vi "Func-엑셀 데이터를 그래프로 출력.vi"() -> ()   [LabVIEW 2015] (continued)
65\t66.118\n65\t65\t66.122\n65\t65\t66.121\n65\t65\t66.127\n65\t65\t66.131\n65\t65\t66.133\n65\t65\t66.137\n65\t65\t66.142\n65\t65\t66.146\n65\t65\t66.148\n65\t65\t66.151\n65\t65\t66.159\n65\t65\t66.161\n65\t65\t66.172\n65\t65\t66.18\n65\t65\t66.186\n65\t65\t66.193\n65\t65\t66.193\n65\t65\t66.2\n65\t65\t66.203\n65\t65\t66.207\n65\t65\t66.213\n65\t65\t66.22\n65\t65\t66.229\n65\t65\t66.235\n65\t65\t66.24\n65\t65\t66.241\n65\t65\t66.25\n65\t65\t66.253\n65\t65\t66.255\n65\t65\t66.258\n65\t65\t66.26\n65\t65\t66.269\n65\t65\t66.273\n65\t65\t66.275\n65\t65\t66.28\n65\t65\t66.287\n65\t65\t66.292\n65\t65\t66.293\n65\t65\t66.298\n65\t65\t66.306\n65\t65\t66.312\n65\t65\t66.318\n65\t65\t66.323\n65\t65\t66.334\n65\t65\t66.34\n65\t65\t66.345\n65\t65\t66.355\n65\t65\t66.36\n65\t65\t66.363\n65\t65\t66.37\n65\t65\t66.37\n65\t65\t66.371\n65\t65\t66.371\n65\t65\t66.377\n65\t65\t66.384\n65\t65\t66.388\n65\t65\t66.393\n65\t65\t66.4\n65\t65\t66.405\n65\t65\t66.407\n65\t65\t66.409\n65\t65\t66.416\n65\t65\t66.424\n65\t65\t66.427\n65\t65\t66.436\n65\t65\t66.44\n65\t65\t66.444\n65\t65\t66.446\n65\t65\t66.448\n65\t65\t66.452\n65\t65\t66.458\n65\t65\t66.463\n65\t65\t66.471\n65\t65\t66.475\n65\t65\t66.484\n65\t65\t66.493\n65\t65\t66.497\n65\t65\t66.506\n65\t65\t66.516\n65\t65\t66.522\n65\t65\t66.525\n65\t65\t66.527\n65\t65\t66.532\n65\t65\t66.532\n65\t65\t66.532\n65\t65\t66.535\n65\t65\t66.545\n65\t65\t66.546\n65\t65\t66.548\n65\t65\t66.55\n65\t65\t66.56\n65\t65\t66.568\n65\t65\t66.571\n65\t65\t66.577\n65\t65\t66.586\n65\t65\t66.591\n65\t65\t66.592\n65\t65\t66.593\n65\t65\t66.597\n65\t65\t66.599\n65\t65\t66.601\n65\t65\t66.609\n65\t65\t66.611\n65\t65\t66.614\n65\t65\t66.619\n65\t65\t66.624\n65\t65\t66.627\n65\t65\t66.629\n65\t65\t66.635\n65\t65\t66.641\n65\t65\t66.645\n65\t65\t66.649\n65\t65\t66.66\n65\t65\t66.666\n65\t65\t66.668\n65\t65\t66.673\n65\t65\t66.68\n65\t65\t66.687\n65\t65\t66.694\n65\t65\t66.699\n65\t65\t66.707\n65\t65\t66.713\n65\t65\t66.717\n65\t65\t66.724\n65\t65\t66.723\n65\t65\t66.73\n65\t65\t66.73\n65\t65\t66.733\n65\t65\t66.736\n65\t65\t66.741\n65\t65\t66.746\n65\t65\t66.747\n65\t65\t66.758\n65\t65\t66.761\n65\t65\t66.761\n65\t65\t66.764\n65\t65\t66.766\n65\t65\t66.773\n65\t65\t66.779\n65\t65\t66.783\n65\t65\t66.79\n65\t65\t66.798\n65\t65\t66.802\n65\t65\t66.804\n65\t65\t66.807\n65\t65\t66.813\n65\t65\t66.818\n65\t65\t66.823\n65\t65\t66.825\n65\t65\t66.827\n65\t65\t66.834\n65\t65\t66.835\n65\t65\t66.84\n65\t65\t66.846\n65\t65\t66.852\n65\t65\t66.862\n65\t65\t66.866\n65\t65\t66.872\n65\t65\t66.879\n65\t65\t66.879\n65\t65\t66.884\n65\t65\t66.891\n65\t65\t66.893\n65\t65\t66.898\n65\t65\t66.9\n65\t65\t66.906\n65\t65\t66.909\n65\t65\t66.909\n65\t65\t66.914\n65\t65\t66.918\n65\t65\t66.925\n65\t65\t66.93\n65\t65\t66.934\n65\t65\t66.939\n65\t65\t66.943\n65\t65\t66.946\n65\t65\t66.948\n65\t65\t66.952\n65\t65\t66.955\n65\t65\t66.958\n65\t65\t66.963\n65\t65\t66.971\n65\t65\t66.976\n65\t65\t66.977\n65\t65\t66.984\n65\t65\t66.988\n65\t65\t66.988\n65\t65\t66.993\n65\t65\t66.998\n65\t65\t67.005\n65\t65\t67.014\n65\t65\t67.021\n65\t65\t67.025\n65\t65\t67.028\n65\t65\t67.029\n65\t65\t67.029\n65\t65\t67.031\n65\t65\t67.033\n65\t65\t67.043\n65\t65\t67.049\n65\t65\t67.05\n65\t65\t67.058\n65\t65\t67.064\n65\t65\t67.069\n65\t65\t67.074\n65\t65\t67.078\n65\t65\t67.087\n65\t65\t67.09\n65\t65\t67.091\n65\t65\t67.091\n65\t65\t67.091\n65\t65\t67.091\n65\t65\t67.093\n65\t65\t67.101\n65\t65\t67.104\n65\t65\t67.113\n65\t65\t67.118\n65\t65\t67.126\n65\t65\t67.129\n65\t65\t67.13\n65\t65\t67.136\n65\t65\t67.139\n65\t65\t67.147\n65\t65\t67.148\n65\t65\t67.155\n65\t65\t67.162\n65\t65\t67.166\n65\t65\t67.175\n65\t65\t67.179\n65\t65\t67.184\n65\t65\t67.187\n65\t65\t67.189\n65\t65\t67.19\n65\t65\t67.191\n65\t65\t67.194\n65\t65\t67.197\n65\t65\t67.204\n65\t65\t67.209\n65\t65\t67.216\n65\t65\t67.221\n65\t65\t67.224\n65\t65\t67.231\n65\t65\t67.232\n65\t65\t67.234\n65\t65\t67.236\n65\t65\t67.239\n65\t65\t67.243\n65\t65\t67.243\n65\t65\t67.248\n65\t65\t67.254\n65\t65\t67.262\n65\t65\t67.264\n65\t65\t67.268\n65\t65\t67.28\n65\t65\t67.285\n65\t65\t67.289\n65\t65\t67.292\n65\t65\t67.298\n65\t65\t67.304\n65\t65\t67.303\n65\t65\t67.308\n65\t65\t67.311\n65\t65\t67.312\n65\t65\t67.317\n65\t65\t67.318\n65\t65\t67.326\n65\t65\t67.332\n65\t65\t67.338\n65\t65\t67.342\n65\t65\t67.347\n65\t65\t67.353\n65\t65\t67.352\n65\t65\t67.352\n65\t65\t67.352\n65\t65\t67.356\n65\t65\t67.357\n65\t65\t67.36\n65\t65\t67.363\n65\t65\t67.372\n65\t65\t67.377\n65\t65\t67.382\n65\t65\t67.388\n65\t65\t67.391\n65\t65\t67.396\n65\t65\t67.399\n65\t65\t67.399\n65\t65\t67.4\n65\t65\t67.406\n65\t65\t67.412\n65\t65\t67.414\n65\t65\t67.417\n65\t65\t67.423\n65\t65\t67.428\n65\t65\t67.429\n65\t65\t67.433\n65\t65\t67.437\n65\t65\t67.445\n65\t65\t67.448\n65\t65\t67.451\n65\t65\t67.454\n65\t65\t67.456\n65\t65\t67.458\n65\t65\t67.458\n65\t65\t67.461\n65\t65\t67.47\n65\t65\t67.475\n65\t65\t67.479\n65\t65\t67.48\n65\t65\t67.486\n65\t65\t67.489\n65\t65\t67.495\n65\t65\t67.498\n65\t65\t67.504\n65\t65\t67.508\n65\t65\t67.513\n65\t65\t67.515\n65\t65\t67.52\n65\t65\t67.52\n65\t65\t67.516\n65\t65\t67.523\n65\t65\t67.525\n65\t65\t67.526\n65\t65\t67.528\n65\t65\t67.533\n65\t65\t67.543\n65\t65\t67.549\n65\t65\t67.554\n65\t65\t67.559\n65\t65\t67.563\n65\t65\t67.564\n65\t65\t67.565\n65\t65\t67.567\n65\t65\t67.571\n65\t65\t67.58\n65\t65\t67.583\n65\t65\t67.588\n65\t65\t67.594\n65\t65\t67.6\n65\t65\t67.599\n65\t65\t67.6\n65\t65\t67.603\n65\t65\t67.61\n65\t65\t67.613\n65\t65\t67.613\n65\t65\t67.62\n65\t65\t67.62\n65\t65\t67.624\n65\t65\t67.631\n65\t65\t67.638\n65\t65\t67.642\n65\t65\t67.646\n65\t65\t67.65\n65\t65\t67.654\n65\t65\t67.651\n65\t65\t67.652\n65\t65\t67.654\n65\t65\t67.661\n65\t65\t67.667\n65\t65\t67.671\n65\t65\t67.677\n65\t65\t67.678\n65\t65\t67.681\n65\t65\t67.683\n65\t65\t67.683\n65\t65\t67.685\n65\t65\t67.692\n65\t65\t67.697\n65\t65\t67.702\n65\t65\t67.711\n65\t65\t67.717\n65\t65\t67.721\n65\t65\t67.724\n65\t65\t67.728\n65\t65\t67.73\n65\t65\t67.73\n65\t65\t67.731\n65\t65\t67.738\n65\t65\t67.738\n65\t65\t67.741\n65\t65\t67.743\n65\t65\t67.748\n65\t65\t67.75\n65\t65\t67.748\n65\t65\t67.752\n65\t65\t67.756\n65\t65\t67.759\n65\t65\t67.762\n65\t65\t67.768\n65\t65\t67.773\n65\t65\t67.778\n65\t65\t67.779\n65\t65\t67.788\n65\t65\t67.793\n65\t65\t67.798\n65\t65\t67.805\n65\t65\t67.806\n65\t65\t67.809\n65\t65\t67.808\n65\t65\t67.807\n65\t65\t67.807\n65\t65\t67.806\n65\t65\t67.811\n65\t65\t67.818\n65\t65\t67.822\n65\t65\t67.824\n65\t65\t67.83\n65\t65\t67.833\n65\t65\t67.835\n65\t65\t67.841\n65\t65\t67.846\n65\t65.01\t67.852\n65\t65.01\t67.855\n65\t65\t67.856\n65\t65.01\t67.859\n65\t65\t67.861\n65\t65\t67.864\n65\t65\t67.867\n65\t65.01\t67.872\n65\t65.01\t67.877\n65\t65.01\t67.882\n65\t65.01\t67.888\n65\t65\t67.89\n65\t65.01\t67.894\n65\t65.01\t67.893\n65\t65.01\t67.896\n65\t65.01\t67.899\n65\t65.01\t67.896\n65\t65.01\t67.896\n65\t65\t67.903\n65\t65\t67.909\n65\t65\t67.911\n65\t65\t67.912\n65\t65\t67.918\n65\t65\t67.924\n65\t65\t67.928\n65\t65\t67.931\n65\t65\t67.935\n65\t65\t67.94\n65\t65\t67.941\n65\t65\t67.943\n65\t65\t67.945\n65\t65\t67.946\n65\t65\t67.948\n65\t65\t67.951\n65\t65\t67.957\n65\t65\t67.962\n65\t65\t67.965\n65\t65\t67.967\n65\t65\t67.974\n65\t65\t67.983\n65\t65\t67.987\n65\t65\t67.986\n65\t65\t67.993\n65\t65\t67.999\n65\t65\t68.003\n65\t65\t68.001\n65\t65\t68.005\n65\t65\t68.009\n65\t65\t68.007\n65\t65\t68.005\n65\t65\t68.007\n65\t65\t68.011\n65\t65\t68.011\n65\t65\t68.02\n65\t65\t68.024\n65\t65\t68.034\n65\t65\t68.034\n65\t65\t68.037\n65\t65\t68.044\n65\t65\t68.043\n65\t65\t68.045\n65\t65\t68.048\n65\t65\t68.053\n65\t65\t68.059\n65\t65\t68.06\n65\t65\t68.066\n65\t65\t68.069\n65\t65\t68.071\n65\t65\t68.075\n65\t65\t68.077\n65\t65\t68.081\n65\t65\t68.08\n65\t65\t68.084\n65\t65\t68.089\n65\t65\t68.089\n65\t65\t68.091\n65\t65\t68.09\n65\t65\t68.094\n65\t65\t68.094\n65\t65\t68.092\n65\t65\t68.094\n65\t65\t68.097\n65\t65\t68.103\n65\t65\t68.107\n65\t65\t68.112\n65\t65\t68.114\n65\t65\t68.119\n65\t65\t68.123\n65\t65\t68.122\n65\t65\t68.121\n65\t65\t68.129\n65\t65\t68.139\n65\t65\t68.142\n65\t65\t68.145\n65\t65\t68.149\n65\t65\t68.155\n65\t65\t68.154\n65\t65\t68.151\n65\t65\t68.154\n65\t65\t68.159\n65\t65\t68.16\n65\t65\t68.165\n65\t65\t68.173\n65\t65\t68.177\n65\t65\t68.177\n65\t65\t68.181\n65\t65\t68.185\n65\t65\t68.187\n65\t65\t68.187\n65\t65\t68.189\n65\t65\t68.194\n65\t65\t68.196\n65\t65\t68.199\n65\t65\t68.206\n65\t65\t68.211\n65\t65\t68.214\n65\t65\t68.219\n65\t65\t68.22\n65\t65\t68.223\n65\t65\t68.227\n65\t65\t68.229\n65\t65\t68.228\n65\t65\t68.23\n65\t65\t68.235\n65\t65\t68.239\n65\t65\t68.239\n65\t65\t68.245\n65\t65\t68.254\n65\t65\t68.255\n65\t65\t68.257\n65\t65\t68.257\n65\t65\t68.261\n65\t65\t68.26\n65\t65\t68.262\n65\t65\t68.265\n65\t65\t68.268\n65\t65\t68.273\n65\t65\t68.274\n65\t65\t68.276\n65\t65\t68.279\n65\t65\t68.286\n65\t65\t68.287\n65\t65\t68.292\n65\t65\t68.297\n65\t65\t68.301\n65\t65\t68.302\n65\t65\t68.304\n65\t65\t68.309\n65\t65\t68.309\n65\t65\t68.31\n65\t65\t68.314\n65\t65\t68.317\n65\t65\t68.316\n65\t65\t68.321\n65\t65\t68.325\n65\t65\t68.33\n65\t65\t68.337\n65\t65\t68.338\n65\t65\t68.341\n65\t65\t68.344\n65\t65\t68.346\n65\t65\t68.349\n65\t65\t68.345\n65\t65\t68.348\n65\t65\t68.351\n65\t65\t68.351\n65\t65\t68.352\n65\t65\t68.353\n65\t65\t68.36\n65\t65\t68.36\n65\t65\t68.364\n65\t65\t68.37\n65\t65\t68.374\n65\t65\t68.38\n65\t65\t68.378\n65\t65\t68.383\n65\t65\t68.388\n65\t65\t68.39\n65\t65\t68.39\n65\t65\t68.391\n65\t65\t68.396\n65\t65\t68.396\n65\t65\t68.399\n65\t65\t68.403\n65\t65\t68.407\n65\t65\t68.409\n65\t65\t68.412\n65\t65\t68.409\n65\t65\t68.409\n65\t65\t68.411\n65\t65\t68.411\n65\t65\t68.418\n65\t65\t68.42\n65\t65\t68.428\n65\t65\t68.436\n65\t65\t68.437\n65\t65\t68.441\n65\t65\t68.441\n65\t65\t68.448\n65\t65\t68.453\n65\t65\t68.451\n65\t65\t68.451\n65\t65\t68.455\n65\t65\t68.456\n65\t65\t68.452\n65\t65\t68.455\n65\t65\t68.458\n65\t65\t68.465\n65\t65\t68.467\n65\t65\t68.471\n65\t65\t68.475\n65\t65\t68.476\n65\t65\t68.479\n65\t65\t68.481\n65\t65\t68.484\n65\t65\t68.485\n65\t65\t68.493\n65\t65\t68.498\n65\t65\t68.497\n65\t65\t68.501\n65\t65\t68.506\n65\t65\t68.508\n65\t65\t68.507\n65\t65\t68.504\n65\t65\t68.51\n65\t65\t68.509\n65\t65\t68.51\n65\t65\t68.514\n65\t65\t68.516\n65\t65\t68.523\n65\t65\t68.527\n65\t65\t68.527\n65\t65\t68.527\n65\t65\t68.532\n65\t65\t68.536\n65\t65\t68.536\n65\t65\t68.542\n65\t65\t68.548\n65\t65\t68.555\n65\t65\t68.556\n65\t65\t68.559\n65\t65\t68.56\n65\t65\t68.558\n65\t65\t68.559\n65\t65\t68.56\n65\t65\t68.564\n65\t65\t68.565\n65\t65\t68.57\n65\t65\t68.574\n65\t65\t68.58\n65\t65\t68.58\n65\t65\t68.582\n65\t65\t68.586\n65\t65\t68.59\n65\t65\t68.589\n65\t65\t68.591\n65\t65\t68.595\n65\t65\t68.598\n65\t65\t68.598\n65\t65\t68.599\n65\t65\t68.603\n65\t65\t68.601\n65\t65\t68.606\n65\t65\t68.606\n65\t65\t68.611\n65\t65\t68.613\n65\t65\t68.614\n65\t65\t68.62\n65\t65\t68.623\n65\t65\t68.627\n65\t65\t68.624\n65\t65\t68.628\n65\t65\t68.628\n65\t65\t68.626\n65\t65\t68.627\n65\t65\t68.63\n65\t65\t68.637\n65\t65\t68.638\n65\t65\t68.643\n65\t65\t68.647\n65\t65\t68.648\n65\t65\t68.652\n65\t65\t68.656\n65\t65\t68.66\n65\t65\t68.664\n65\t65\t68.669\n65\t65\t68.671\n65\t65\t68.672\n65\t65\t68.671\n65\t65\t68.671\n65\t65\t68.671\n65\t65\t68.673\n65\t65\t68.68\n65\t65\t68.68\n65\t65\t68.687\n65\t65\t68.693\n65\t65\t68.698\n65\t65\t68.696\n65\t65\t68.695\n65\t65\t68.697\n65\t65\t68.698\n65\t65\t68.698\n65\t65\t68.701\n65\t65\t68.709\n65\t65\t68.713\n65\t65\t68.717\n65\t65\t68.718\n65\t65\t68.719\n65\t65\t68.72\n65\t65\t68.718\n65\t65\t68.718\n65\t65\t68.72\n65\t65\t68.722\n65\t65\t68.721\n65\t65\t68.725\n65\t65\t68.731\n65\t65\t68.736\n65\t65\t68.739\n65\t65\t68.74\n65\t65\t68.747\n65\t65\t68.749\n65\t65\t68.749\n65\t65\t68.75\n65\t65\t68.754\n65\t65\t68.757\n65\t65\t68.757\n65\t65\t68.758\n65\t65\t68.762\n65\t65\t68.767\n65\t65\t68.767\n65\t65\t68.77\n65\t65\t68.773\n65\t65\t68.777\n65\t65\t68.78\n65\t65\t68.78\n65\t65\t68.783\n65\t65\t68.784\n65\t65\t68.788\n65\t65\t68.786\n65\t65\t68.787\n65\t65\t68.789\n65\t65\t68.788\n65\t65\t68.784\n65\t65\t68.786\n65\t65\t68.787\n65\t65\t68.79\n65\t65\t68.793\n65\t65\t68.8\n65\t65\t68.809\n65\t65\t68.811\n65\t65\t68.817\n65\t65\t68.82\n65\t65\t68.82\n65\t65\t68.82\n65\t65\t68.819\n65\t65\t68.82\n65\t65\t68.822\n65\t65\t68.825\n65\t65\t68.827\n65\t65\t68.829\n65\t65\t68.836\n65\t65\t68.838\n65\t65\t68.838\n65\t65\t68.843\n65\t65\t68.844\n65\t65\t68.848\n65\t65\t68.849\n65\t65\t68.85\n65\t65\t68.85\n65\t65\t68.85\n65\t65\t68.852\n65\t65\t68.857\n65\t65\t68.859\n65\t65\t68.863\n65\t65\t68.868\n65\t65\t68.87\n65\t65\t68.873\n65\t65\t68.87\n65\t65\t68.875\n65\t65\t68.878\n65\t65\t68.883\n65\t65\t68.884\n65\t65\t68.886\n65\t65\t68.889\n65\t65\t68.887\n65\t65\t68.889\n65\t65\t68.893\n65\t65\t68.894\n65\t65\t68.899\n65\t65\t68.903\n65\t65\t68.907\n65\t65\t68.908\n65\t65\t68.907\n65\t65\t68.911\n65\t65\t68.913\n65\t65\t68.914\n65\t65\t68.918\n65\t65\t68.923\n65\t65\t68.924\n65\t65\t68.927\n65\t65\t68.929\n65\t65\t68.931\n65\t65\t68.932\n65\t65\t68.934\n65\t65\t68.934\n65\t65\t68.935\n65\t65\t68.937\n65\t65\t68.94\n65\t65\t68.943\n65\t65\t68.944\n65\t65\t68.95\n65\t65\t68.955\n65\t65\t68.957\n65\t65\t68.955\n65\t65\t68.958\n65\t65\t68.961\n65\t65\t68.959\n65\t65\t68.954\n65\t65\t68.957\n65\t65\t68.96\n65\t65\t68.964\n65\t65\t68.965\n65\t65\t68.973\n65\t65\t68.977\n65\t65\t68.975\n65\t65\t68.977\n65\t65\t68.977\n65\t65\t68.978\n65\t65\t68.974\n65\t65\t68.977\n65\t65\t68.98\n65\t65\t68.982\n65\t65\t68.987\n65\t65\t68.993\n65\t65\t68.996\n65\t65\t68.998\n65\t65\t69.001\n65\t65\t69\n65\t65\t69.002\n65\t65\t69.002\n65\t65\t69.001\n65\t65\t69.005\n65\t65\t69.003\n65\t65\t69.007\n65\t65\t69.003\n65\t65\t69.004\n65\t65\t69.01\n65\t65\t69.014\n65\t65\t69.02\n65\t65\t69.021\n65\t65\t69.029\n65\t65\t69.03\n65\t65\t69.029\n65\t65\t69.031\n65\t65\t69.03\n65\t65\t69.032\n65\t65\t69.033\n65\t65\t69.034\n65\t65\t69.038\n65\t65\t69.037\n65\t65\t69.046\n65\t65\t69.047\n65\t65\t69.045\n65\t65\t69.046\n65\t65\t69.046\n65\t65\t69.051\n65\t65\t69.049\n65\t65\t69.05\n65\t65\t69.057\n65\t65\t69.062\n65\t65\t69.066\n65\t65\t69.065\n65\t65\t69.066\n65\t65\t69.067\n65\t65\t69.069\n65\t65\t69.069\n65\t65\t69.068\n65\t65\t69.071\n65\t65\t69.073\n65\t65\t69.075\n65\t65\t69.077\n65\t65\t69.077\n65\t65\t69.08\n65\t65\t69.084\n65\t65\t69.088\n65\t65\t69.091\n65\t65\t69.093\n65\t65\t69.097\n65\t65\t69.098\n65\t65\t69.102\n65\t65\t69.101\n65\t65\t69.104\n65\t65\t69.104\n65\t65\t69.106\n65\t65\t69.111\n65\t65\t69.11\n65\t65\t69.113\n65\t65\t69.115\n65\t65\t69.118\n65\t65\t69.12\n65\t65\t69.117\n65\t65\t69.117\n65\t65\t69.121\n65\t65\t69.122\n65\t65\t69.123\n65\t65\t69.121\n65\t65\t69.125\n65\t65\t69.13\n65\t65\t69.13\n65\t65\t69.135\n65\t65\t69.136\n65\t65\t69.138\n65\t65\t69.144\n65\t65\t69.146\n65\t65\t69.146\n65\t65\t69.149\n65\t65\t69.151\n65\t65\t69.149\n65\t65\t69.15\n65\t65\t69.148\n65\t65\t69.152\n65\t65\t69.15\n65\t65\t69.15\n65\t65\t69.153\n65\t65\t69.155\n65\t65\t69.16\n65\t65\t69.164\n65\t65\t69.167\n65\t65\t69.171\n65\t65\t69.176\n65\t65\t69.171\n65\t65\t69.173\n65\t65\t69.176\n65\t65\t69.177\n65\t65\t69.18\n65\t65\t69.182\n65\t65\t69.186\n65\t65\t69.19\n65\t65\t69.191\n65\t65\t69.194\n65\t65\t69.194\n65\t65\t69.198\n65\t65\t69.201\n65\t65\t69.202\n65\t65\t69.204\n65\t65\t69.204\n65\t65\t69.21\n65\t65\t69.21\n65\t65\t69.209\n65\t65\t69.209\n65\t65\t69.209\n65\t65\t69.207\n65\t65\t69.209\n65\t65\t69.215\n65\t65\t69.22\n65\t65\t69.221\n65\t65\t69.225\n65\t65\t69.229\n65\t65\t69.233\n65\t65\t69.232\n65\t65\t69.233\n65\t65\t69.238\n65\t65\t69.238\n65\t65\t69.242\n65\t65\t69.241\n65\t65\t69.244\n65\t65\t69.241\n65\t65\t69.243\n65\t65\t69.249\n65\t65\t69.246\n65\t65\t69.246\n65\t65\t69.245\n65\t65\t69.25\n65\t65\t69.254\n65\t65\t69.254\n65\t65\t69.259\n65\t65\t69.262\n65\t65\t69.265\n65\t65\t69.263\n65\t65\t69.262\n65\t65\t69.264\n65\t65\t69.266\n65\t65\t69.266\n65\t65\t69.266\n65\t65\t69.268\n65\t65\t69.27\n65\t65\t69.273\n65\t65\t69.273\n65\t65\t69.273\n65\t65\t69.279\n65\t65\t69.281\n65\t65\t69.279\n65\t65\t69.275\n65\t65\t69.276\n65\t65\t69.282\n65\t65\t69.28\n65\t65\t69.285\n65\t65\t69.289\n65\t65\t69.294\n65\t65\t69.297\n65\t65\t69.298\n65\t65\t69.305\n65\t65\t69.304\n65\t65\t69.305\n65\t65\t69.308\n65\t65\t69.308\n65\t65\t69.311\n65\t65\t69.308\n65\t65\t69.312\n65\t65\t69.317\n65\t65\t69.314\n65\t65\t69.316\n65\t65\t69.316\n65\t65\t69.32\n65\t65\t69.321\n65\t65\t69.318\n65\t65\t69.324\n65\t65\t69.323\n65\t65\t69.329\n65\t65\t69.331\n65\t65\t69.33\n65\t65\t69.337\n65\t65\t69.338\n65\t65\t69.34\n65\t65\t69.337\n65\t65\t69.338\n65\t65\t69.346\n65\t65\t69.345\n65\t65\t69.347\n65\t65\t69.348\n65\t65\t69.349\n65\t65\t69.349\n65\t65\t69.349\n65\t65\t69.35\n65\t65\t69.352\n65\t65\t69.356\n65\t65\t69.358\n65\t65\t69.364\n65\t65\t69.364\n65\t65\t69.365\n65\t65\t69.367\n65\t65\t69.368\n65\t65\t69.371\n65\t65\t69.368\n65\t65\t69.373\n65\t65\t69.376\n65\t65\t69.379\n65\t65\t69.38\n65\t65\t69.385\n65\t65\t69.386\n65\t65\t69.384\n65\t65\t69.387\n65\t65\t69.382\n65\t65\t69.383\n65\t65\t69.38\n65\t65\t69.385\n65\t65\t69.387\n65\t65\t69.389\n65\t65\t69.393\n65\t65\t69.399\n65\t65\t69.403\n65\t65\t69.4\n65\t65\t69.4\n65\t65\t69.4\n65\t65\t69.402\n65\t65\t69.403\n65\t65\t69.405\n65\t65\t69.408\n65\t65\t69.409\n65\t65\t69.409\n65\t65\t69.411\n65\t65\t69.407\n65\t65\t69.404\n65\t65\t69.403\n65\t65\t69.405\n65\t65\t69.411\n65\t65\t69.41\n65\t65\t69.411\n65\t65\t69.42\n65\t65\t69.422\n65\t65\t69.426\n65\t65\t69.428\n65\t65\t69.43\n65\t65\t69.434\n65\t65\t69.433\n65\t65\t69.435\n65\t65\t69.432\n65\t65\t69.434\n65\t65\t69.437\n65\t65\t69.439\n65\t65\t69.44\n65\t65\t69.444\n65\t65\t69.448\n65\t65\t69.447\n65\t65\t69.442\n65\t65\t69.445\n65\t65\t69.446\n65\t65\t69.447\n65\t65\t69.452\n65\t65\t69.452\n65\t65\t69.454\n65\t65\t69.456\n65\t65\t69.457\n65\t65\t69.457\n65\t65\t69.455\n65\t65\t69.458\n65\t65\t69.463\n65\t65\t69.468\n65\t65\t69.467\n65\t65\t69.472\n65\t65\t69.475\n65\t65\t69.474\n65\t65\t69.468\n65\t65\t69.468\n65\t65\t69.475\n65\t65\t69.476\n65\t65\t69.475\n65\t65\t69.475\n65\t65\t69.479\n65\t65\t69.479\n65\t65\t69.479\n65\t65\t69.482\n65\t65\t69.486\n65\t65\t69.49\n65\t65\t69.491\n65\t65\t69.494\n65\t65\t69.496\n65\t65\t69.497\n65\t65\t69.5\n65\t65\t69.502\n65\t65\t69.506\n65\t65\t69.504\n65\t65\t69.502\n65\t65\t69.503\n65\t65\t69.5\n65\t65\t69.502\n65\t65\t69.502\n65\t65\t69.507\n65\t65\t69.507\n65\t65\t69.507\n65\t65\t69.507\n65\t65\t69.509\n65\t65\t69.506\n65\t65\t69.509\n65\t65\t69.512\n65\t65\t69.515\n65\t65\t69.516\n65\t65\t69.52\n65\t65\t69.522\n65\t65\t69.525\n65\t65\t69.527\n65\t65\t69.526\n65\t65\t69.53\n65\t65\t69.53\n65\t65\t69.532\n65\t65\t69.53\n65\t65\t69.531\n65\t65\t69.533\n65\t65\t69.536\n65\t65\t69.541\n65\t65\t69.544\n65\t65\t69.547\n65\t65\t69.548\n65\t65\t69.552\n65\t65\t69.55\n65\t65\t69.548\n65\t65\t69.55\n65\t65\t69.551\n65\t65\t69.549\n65\t65\t69.548\n65\t65\t69.55\n65\t65\t69.555\n65\t65\t69.554\n65\t65\t69.559\n65\t65\t69.562\n65\t65\t69.567\n65\t65\t69.567\n65\t65\t69.565\n65\t65\t69.566\n65\t65\t69.566\n65\t65\t69.564\n65\t65\t69.564\n65\t65\t69.564\n65\t65\t69.568\n65\t65\t69.571\n65\t65\t69.573\n65\t65\t69.579\n65\t65\t69.579\n65\t65\t69.579\n65\t65\t69.577\n65\t65\t69.575\n65\t65\t69.579\n65\t65\t69.578\n65\t65\t69.58\n65\t65\t69.584\n65\t65\t69.589\n65\t65\t69.592\n65\t65\t69.591\n65\t65\t69.595\n65\t65\t69.597\n65\t65\t69.597\n65\t65\t69.597\n65\t65\t69.599\n65\t65\t69.601\n65\t65\t69.609\n65\t65\t69.611\n65\t65\t69.609\n65\t65\t69.609\n65\t65\t69.611\n65\t65\t69.613\n65\t65\t69.609\n65\t65\t69.608\n65\t65\t69.607\n65\t65\t69.61\n65\t65\t69.609\n65\t65\t69.605\n65\t65\t69.608\n65\t65\t69.616\n65\t65\t69.619\n65\t65\t69.621\n65\t65\t69.624\n65\t65\t69.629\n65\t65\t69.627\n65\t65\t69.622\n65\t65\t69.623\n65\t65\t69.626\n65\t65\t69.624\n65\t65\t69.623\n65\t65\t69.626\n65\t65\t69.627\n65\t65\t69.629\n65\t65\t69.63\n65\t65\t69.63\n65\t65\t69.634\n65\t65\t69.636\n65\t65\t69.638\n65\t65\t69.638\n65\t65\t69.642\n65\t65\t69.647\n65\t65\t69.648\n65\t65\t69.653\n65\t65\t69.65\n65\t65\t69.653\n65\t65\t69.652\n65\t65\t69.652\n65\t65\t69.654\n65\t65\t69.652\n65
